vi "readRX TEST.vi"() -> ()   [LabVIEW 2019]
uses:
  SPI/SPI Config.ctl
panel:
  out "Data Read":u8[](array[numeric]) format="%08b"
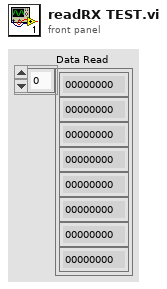
[diagram p1: front panel]
types:
  T1 = typedef "SPI Config.ctl" = cluster{"MXP Port":enum16{"A", "B"}, "Device":enum16{"CAN", "ENC", "IMU1", "IMU2"}, "CPOL":bool}
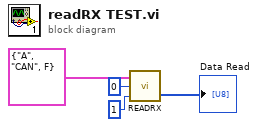
[diagram p0: block diagram]
diagram:
  n1 = call "READRX.vi"("Registers to Read"=u8 1, "Reg. Select"=u8 0, "SPI Config In"=T1 {"MXP Port"=enum."A", "Device"=enum."CAN", "CPOL"=FALSE}) -> ("Data Read"=→"Data Read":u8[])  [unwired: 1 out]
